vi "Make serial number.vi"() -> (1 "Read":string, 2 "serial number":string, 3 "Yearweek":string)   [LabVIEW 2009]
uses:
  Global/Global 1.vi
panel:
  out "F-format string":string
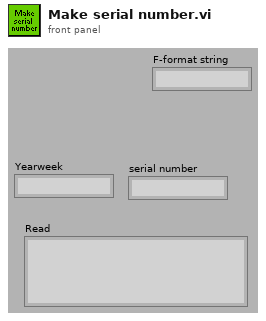
[diagram p1: front panel]
types:
  T1 = enum16{"open", "replace", "create", "open or create", "replace or create", "replace or create with confirmation"}
  T2 = typedef "LVDateTimeRec.ctl" = cluster{"秒数的小数部分":dbl, "秒":i32, "分":i32, "小时":i32, "日":i32, "月":i32, "年":i32, "天数（周）":i32, "天数（年）":i32, "DST":i32}
  T3 = cluster{"serial number":string, "Part number":string, "Revision letter ":string, "Revision counter":string, "Manufature":string, "Year Week":string}
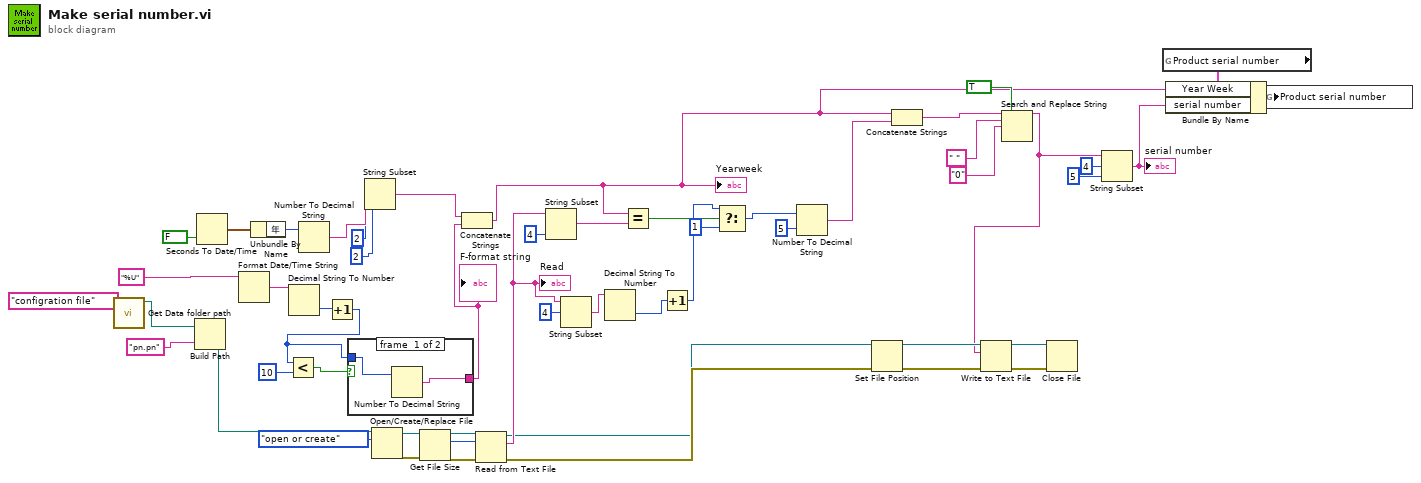
[diagram p0: block diagram]
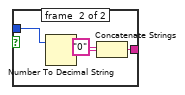
[diagram p2: hidden frame]
diagram:
  n1 = call "Get Data folder path.vi"("Data Path Name"="configration file") -> ("Data Path"=w8:path)  [unwired: 1 in, 9 out]
  n2 = Build Path(base path=w8, name or relative path="pn.pn" ("字符串")) -> (appended path=w44:path)
  n3 = Seconds To Date/Time(to UTC (F)=FALSE ("转换为UTC (F)")) -> (date time rec=w52:T2)  [unwired: 1 out]
  n4 = Format Date/Time String(time format string (%c)="%U" ("时间格式字符串(%c)")) -> (date/time string=w6:string)  [unwired: 2 out]
  n5 = Unbundle By Name(w52) -> ("年"=w51:i32)
  n6 = Decimal String To Number(string=w6) -> (number=w5:i32)  [unwired: 3 out]
  n7 = Number To Decimal String(number=w51) -> (decimal integer string=w49:string)  [unwired: 1 out]
  n8 = Increment(x=w5) -> (x+1=w2:i32)
  n9 = Less?(x=w2, y=10) -> (x < y?=w3:bool)
  n10 = case shown="False" w3 {
    tunnel: w2 -> [w55 w59]
    tunnel: [w54 w56] -> w1
    frame #0 {
      n11 = Number To Decimal String(number=w55) -> (decimal integer string=w54:string)  [unwired: 1 out]
    }
    frame #1 {
      n12 = Number To Decimal String(number=w59) -> (decimal integer string=w58:string)  [unwired: 1 out]
      n13 = Concatenate Strings("0" ("string"), w58) -> (w56:string)
    }
  }
  "F-format string" <- w1
  n14 = String Subset(string=w49, offset (0)=2 ("偏移量(0)"), length (rest)=2 ("长度（剩余）")) -> (substring=w46:string)
  n15 = Open/Create/Replace File(file path (use dialog)=w44, operation (0:open)=T1."open or create" ("操作(0:open)")) -> (refnum out=w43:refnum<file>, error out=w39:errorcluster)  [unwired: 1 in, 4 out]
  n16 = Get File Size(file=w43, error in=w39) -> (refnum out=w42:refnum<file>, size (in bytes)=w41:i64, 0:w40:errorcluster)
  n17 = Concatenate Strings(w46, w1) -> (w13:string)
  "Yearweek" <- w13
  n18 = Read from Text File(file (use dialog)=w42, count=w41, error in=w40) -> (refnum out=w21:refnum<file>, text=w29:string, error out=w24:errorcluster)  [unwired: 2 out]
  "Read" <- w29
  n19 = String Subset(string=w29, length (rest)=4 ("长度（剩余）")) -> (substring=w36:string)  [unwired: 1 out]
  n20 = String Subset(string=w29, offset (0)=4 ("偏移量(0)")) -> (substring=w27:string)  [unwired: 1 out]
  n21 = Decimal String To Number(string=w27) -> (number=w35:i32)  [unwired: 3 out]
  n22 = Equal?(x=w13, y=w36) -> (x = y?=w30:bool)
  n23 = Increment(x=w35) -> (x+1=w34:i32)
  n24 = Select(t=w34, s=w30, f=1) -> (s? t:f=w32:i32)
  n25 = Number To Decimal String(number=w32, width (-)=i16 5 ("宽度(-)")) -> (decimal integer string=w14:string)
  n26 = Set File Position(refnum=w21, error in=w24) -> (refnum out=w22:refnum<file>, error out=w23:errorcluster)  [unwired: 2 out]
  n27 = Concatenate Strings(w13, w14) -> (w20:string)
  n28 = Search and Replace String(replace all?=TRUE ("替换全部？(F)"), input string=w20, search string=" " ("regular expression (\"\")"), replace string="0" ("replace string (\"\")")) -> (result string=w12:string)  [unwired: 1 in, 6 out]
  n29 = Write to Text File(file (use dialog)=w22, text=w12, error in=w23) -> (refnum out=w25:refnum<file>, error out=w26:errorcluster)  [unwired: 2 out]
  n30 = Close File(refnum=w25, error in=w26) -> ()  [unwired: 2 out]
  n31 = String Subset(string=w12, offset (0)=4, length (rest)=5 ("length (rest)")) -> (substring=w9:string)
  "serial number" <- w9
  n32 = global read "Global 1.vi" "Product serial number"() -> (w16:T3)
  n33 = Bundle By Name(cluster=w16, "Year Week"=w13, "serial number"=w9) -> (w15:T3)
  n34 = global write "Global 1.vi" "Product serial number"(w15) -> ()
